vi "movimentacao_cin_inv_bezier_2_com_sensor.vi"() -> ()   [LabVIEW 2017]
doc: "The myRIO Project template acquires acceleration data from the onboard accelerometer and displays the changes of acceleration values in a waveform chart."
uses:
  <vilib>/Analysis/Matrix/Datatypes/RealMatrix.ctl
  <vilib>/myRIO/Instrument Drivers/Onboard IO/I2C/typedefs/I2C User Configuration.ctl
  <vilib>/myRIO/Instrument Drivers/Onboard IO/I2C/typedefs/I2C Transfer Rate.ctl
  <vilib>/myRIO/Instrument Drivers/Onboard IO/PWM/typedefs/PWM Reference.ctl
  <vilib>/myRIO/Common/Instrument Driver Framework/Utilities/typedefs/myRIO Generic Hardware Reference.ctl
  <vilib>/myRIO/Common/Instrument Driver Framework/Utilities/typedefs/Hardware Version Enum.ctl
  <vilib>/myRIO/Common/Instrument Driver Framework/Utilities/typedefs/myRIO v1.0 Reference.ctl
  <vilib>/myRIO/Common/Instrument Driver Framework/Utilities/typedefs/Generic FPGA Reference.ctl
  <vilib>/myRIO/Common/Instrument Driver Framework/myRIO v1.0/PWM/typedefs/PWM Channels Enum.ctl
  <vilib>/myRIO/Instrument Drivers/Onboard IO/PWM/typedefs/PWM Configuration.ctl
  <vilib>/userdefined/High Color/nirio_resource_hc.ctl
  <vilib>/myRIO/Instrument Drivers/Onboard IO/I2C/typedefs/I2C Reference.ctl
  <vilib>/myRIO/Common/Instrument Driver Framework/myRIO v1.0/I2C/typedefs/I2C Channels Enum.ctl
  <vilib>/myRIO/Instrument Drivers/Onboard IO/I2C/typedefs/I2C Configuration.ctl
  <vilib>/myRIO/Common/Instrument Driver Framework/myRIO v1.0/I2C/vis/myRIO v1.1 Open I2C.vi
  <vilib>/myRIO/Common/Instrument Driver Framework/myRIO v1.0/PWM/vis/myRIO v1.1 Open PWM.vi
  <vilib>/myRIO/Common/Instrument Driver Framework/Utilities/vis/Validate Channels.vi
  <vilib>/myRIO/Common/Instrument Driver Framework/myRIO v1.0/I2C/vis/myRIO v1.0 Reserve I2C.vi
  <vilib>/myRIO/Common/Instrument Driver Framework/myRIO v1.0/I2C/vis/myRIO v1.0 Close I2C.vi
  <vilib>/myRIO/Common/Instrument Driver Framework/myRIO v1.0/PWM/vis/myRIO v1.0 Reserve PWM.vi
  <vilib>/myRIO/Instrument Drivers/Onboard IO/PWM/vis/Set Duty Cycle and Frequency.vi
  <vilib>/myRIO/Common/Instrument Driver Framework/myRIO v1.0/PWM/vis/myRIO v1.0 Close PWM.vi
  <vilib>/myRIO/Common/Instrument Driver Framework/myRIO v1.0/I2C/vis/myRIO v1.0 Build MUX Configuration I2C.vi
  <vilib>/myRIO/Common/Instrument Driver Framework/myRIO v1.0/Resource Manager/vis/myRIO v1.0 Reserve Channel List.vi
  <vilib>/myRIO/Common/Instrument Driver Framework/myRIO v1.0/I2C/vis/myRIO v1.0 Unreserve I2C.vi
  <vilib>/myRIO/Common/Instrument Driver Framework/myRIO v1.0/PWM/vis/myRIO v1.0 Build MUX Configuration PWM.vi
  <vilib>/myRIO/Common/Instrument Driver Framework/myRIO v1.0/PWM/vis/myRIO v1.0 Unreserve PWM.vi
  <vilib>/myRIO/Common/Instrument Driver Framework/myRIO v1.0/Resource Manager/vis/myRIO v1.0 Create Configuration List.vi
  <vilib>/myRIO/Common/Instrument Driver Framework/myRIO v1.0/Resource Manager/vis/myRIO v1.0 Reserve Channel.vi
  <vilib>/myRIO/Common/Instrument Driver Framework/myRIO v1.0/Resource Manager/vis/myRIO v1.0 Unreserve Channel.vi
  <vilib>/myRIO/Common/Instrument Driver Framework/myRIO v1.0/Resource Manager/vis/myRIO v1.0 Unreserve Channel List.vi
  <vilib>/myRIO/Common/Instrument Driver Framework/myRIO v1.0/Resource Manager/vis/myRIO v1.0 Build Mutex Name.vi
  <vilib>/Utility/VariantDataType/GetNumericInfo.vi
  <vilib>/Utility/error.llb/Error Cluster From Error Code.vi
  <vilib>/myRIO/Common/Instrument Driver Framework/myRIO v1.0/myRIO v1.1 Open.vi
  <vilib>/myRIO/Common/Instrument Driver Framework/Utilities/vis/IO Manager.vi
  <vilib>/myRIO/Common/Instrument Driver Framework/Utilities/vis/Configuration Manager.vi
  <vilib>/myRIO/Common/Instrument Driver Framework/myRIO v1.0/Resource Manager/vis/myRIO v1.0 Configure IO.vi
  <vilib>/myRIO/Common/Instrument Driver Framework/myRIO v1.0/myRIO v1.0 Close.vi
  <vilib>/myRIO/Common/Instrument Driver Framework/myRIO v1.0/PWM/vis/myRIO v1.0 Write PWM.vi
  <vilib>/myRIO/Common/Instrument Driver Framework/myRIO v1.0/PWM/vis/myRIO v1.0 Shutdown PWM.vi
  <vilib>/myRIO/Common/Instrument Driver Framework/myRIO v1.0/I2C/vis/myRIO v1.0 Configure I2C.vi
  <vilib>/myRIO/Common/Instrument Driver Framework/myRIO v1.0/I2C/vis/myRIO v1.0 Shutdown I2C.vi
  <vilib>/myRIO/Instrument Drivers/Onboard IO/PWM/vis/myRIO PWM Open.xnode
  <vilib>/myRIO/Instrument Drivers/Onboard IO/I2C/vis/myRIO I2C Open.xnode
  <vilib>/myRIO/Instrument Drivers/Onboard IO/PWM/PWM.lvlib
  <vilib>/myRIO/Instrument Drivers/Onboard IO/I2C/I2C.lvlib
  <vilib>/Analysis/Matrix/NI_Matrix.lvlib
panel:
  out "Detectou 2":bool
  out "mean out":dbl
  in  "y":dbl=135.0
  out "PARAR ESTEIRA":bool
  out "reconheceu":bool
  out "Boolean":bool
  out "x .and. y? 2":bool
  out "Detectou":bool
  in  "Duty Cycle Abert 2":dbl=0.08 format="%#_13g"
  out "Local_da_peca":i8
  out "PARAR 2":bool
  out "spreadsheet string":string
  out "error out 2":errorcluster
  out "init status 2":bool
  out "did_timeout 2":bool
  out "dt 2":u32
  out "Waveform Chart 2":u16(graph)
  out "Range (cm)":u16
  out "objeto":bool
  out "distancaia 2":dbl format="%0.2f"
  out "result string":string
  out "iterador":u32
  out "number of rows":i32
  out "matrix":T1
  out "subarray":dbl[](array[numeric])
  out "appended array 2":dbl[](array[numeric])
  out "POS_E_ORIEN_HOME":dbl[](array[numeric])
  out "ANG_POSI_E_ORIEN_HOME":dbl[](array[numeric])
  out "CURRENT POSITIONS OF THE MOTORS":dbl[](array[numeric])
  in  "angulo_garra":dbl(knob) scale=-180.0..180.0
  in  "Duty Cycle Abert":dbl=0.04 format="%#_13g"
  out "Actuator 2":bool
  in  "Actuator":bool
  in  "Conveyor speed (mm/s)":dbl(slide)=200.0 step=1.0 scale=0.0..350.0
  out "indexador":i32
  out "Manipulando":bool
  out "Está em Home":bool
  out "Posicao_desejada":bool
  in  "Home":bool
  in  "error in (no error)":errorcluster
  in  "PARAR":bool
  in  "POSITION VECTOR":dbl[](array[numeric])
  # "ROTINA DE CONTROLE DO PROTÓTIPO DE FMS"
  # "COMANDO DE POSI敲O\nATUAL DOS MOTORES"
  # "OPERATION STATUS"
  # "ÂNGULOS DE JUNTAS"
  # "THETA 1"
  # "MOTOR 1"
  # "HOME"
  # "THETA 2"
  # "MOTOR 2"
  # "POSI敲O DESEJADA"
  # "SCL- CINZA - 32\nSDA - ROXO - 34\nTERRA - BRANCO\nVCC - PRETO"
  # "THETA 3"
  # "MOTOR 3"
  # "OBJETO DETECTADO"
  # "THETA 4"
  # "MOTOR 4"
  # "MANIPULANDO"
  # "THETA 5"
  # "MOTOR 5"
  # "ESTEIRA PARADA"
  # "MOTOR 6"
  # "ATUADOR"
  # "VELOCIDADE DA ESTEIRA (mm/s)"
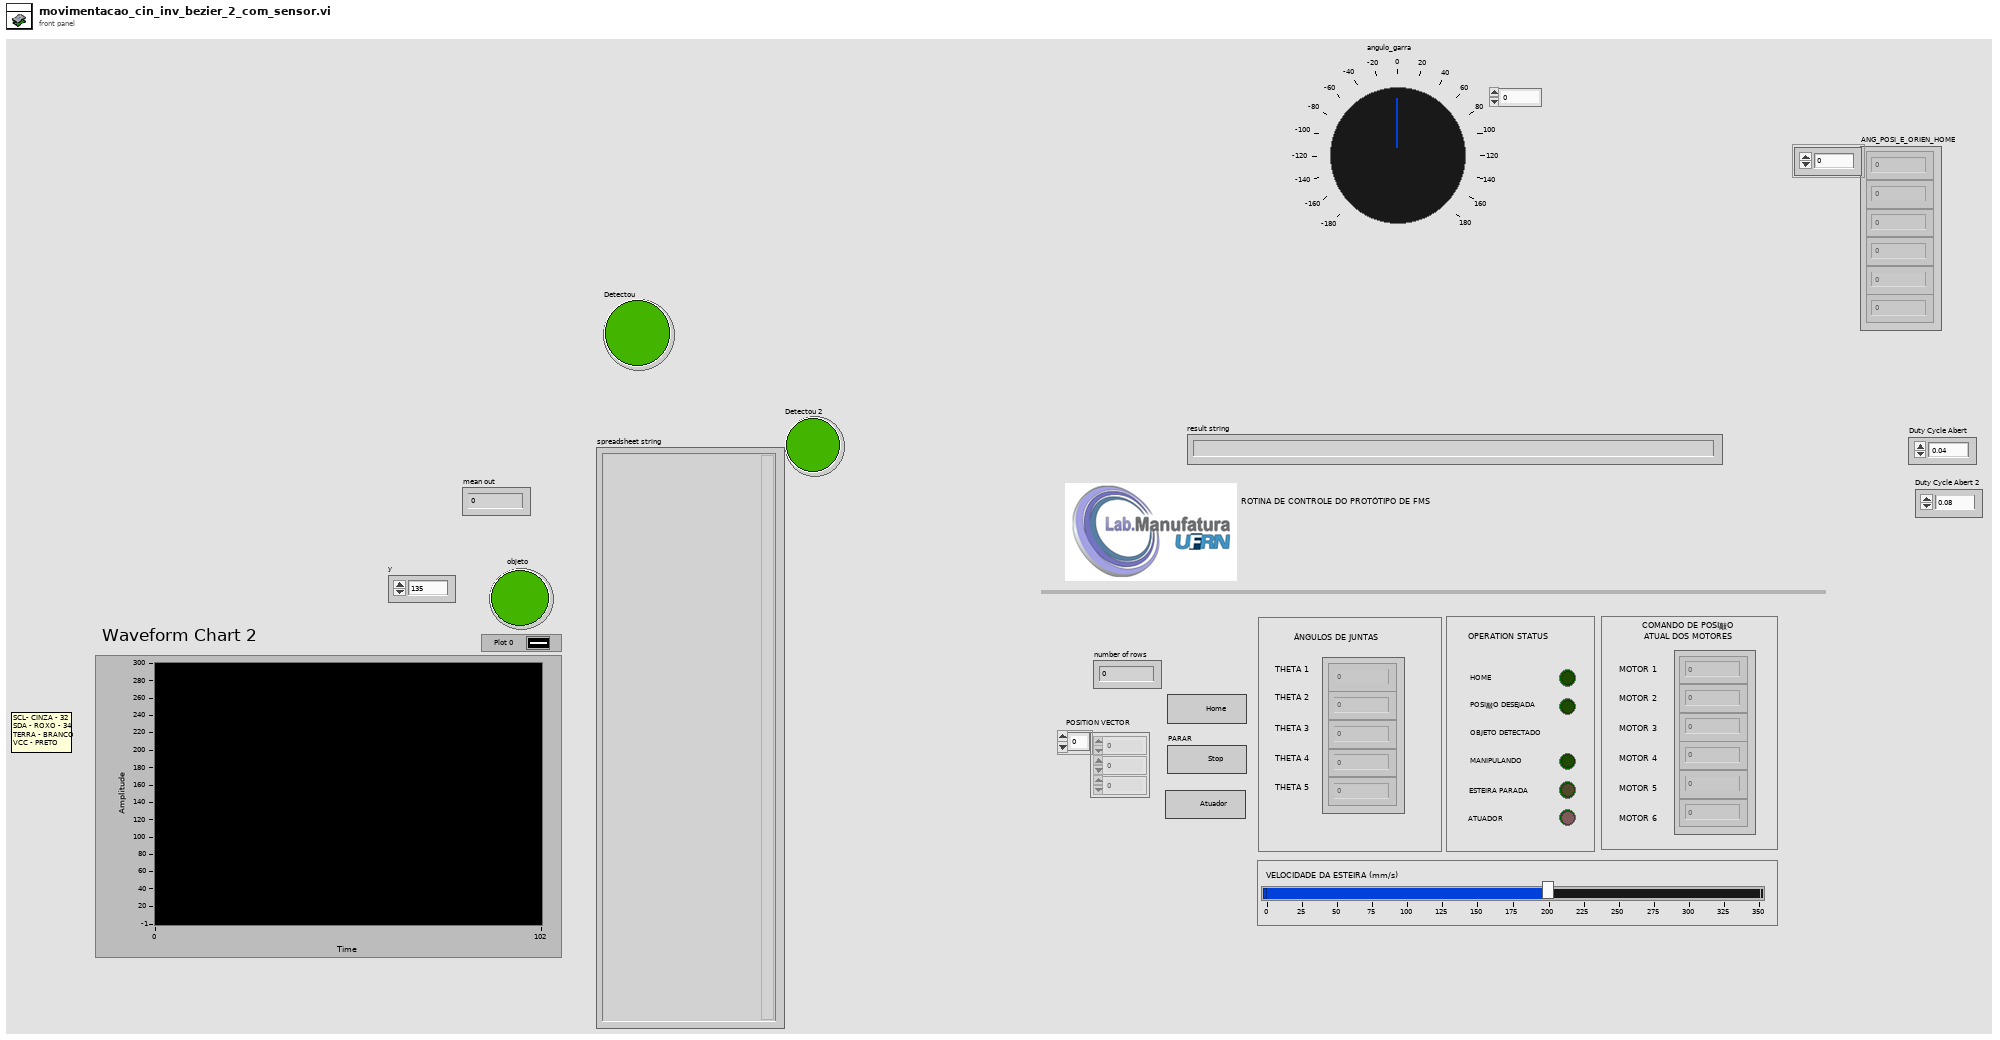
[diagram p1: front panel]
types:
  T1 = typedef "NI_Matrix.lvlib/RealMatrix.ctl" = dbl[][]
  T2 = typedef "I2C.lvlib/I2C User Configuration.ctl" = cluster{"I2C Transfer Rate":T3}
  T3 = typedef "I2C.lvlib/I2C Transfer Rate.ctl" = enum16{"Standard mode (100 kbps)", "Fast mode (400 kbps)"}
  T4 = cluster{"theta 1":dbl, "theta 2":dbl, "theta 3":dbl, "theta5":dbl, "theta4":dbl}
  T5 = typedef "nirio_resource_hc.ctl" = tag
  T6 = typedef "Hardware Version Enum.ctl" = enum16{"Unknown", "myRIO-1900", "myRIO-1950", "roboRIO", "NI ELVIS RIO CM"}
  T7 = typedef "PWM.lvlib/PWM Reference.ctl" = cluster{"myRIO Reference":T8, "PWM Channels Enum":T11, "PWM Configuration":T12}
  T8 = typedef "myRIO Generic Hardware Reference.ctl" = cluster{"myRIO Model":T6, "myRIO Hardware Reference":T9}
  T9 = typedef "myRIO v1.0 Reference.ctl" = cluster{"Generic FPGA Reference":T10, "Allow multiple opens":bool}
  T10 = typedef "Generic FPGA Reference.ctl" = refnum<k20>
  T11 = typedef "PWM Channels Enum.ctl" = enum16{"Not Connected", "C/PWM0", "C/PWM1", "A/PWM0", "A/PWM1", "A/PWM2", "B/PWM0", "B/PWM1", "B/PWM2", "PWM/PWM0", "PWM/PWM1", "PWM/PWM2", "PWM/PWM3", "PWM/PWM4", "PWM/PWM5", "PWM/PWM6", "PWM/PWM7", "PWM/PWM8", "PWM/PWM9"}
  T12 = typedef "PWM.lvlib/PWM Configuration.ctl" = cluster{"Frequency":dbl, "Duty Cycle":dbl}
  T13 = typedef "I2C.lvlib/I2C Reference.ctl" = cluster{"myRIO Reference":T8, "I2C Channels Enum":T14, "I2C Configuration":T15}
  T14 = typedef "I2C Channels Enum.ctl" = enum16{"Not Connected", "A/I2C", "B/I2C", "I2C/I2C"}
  T15 = typedef "I2C.lvlib/I2C Configuration.ctl" = cluster{"I2C Transfer Rate":T3}
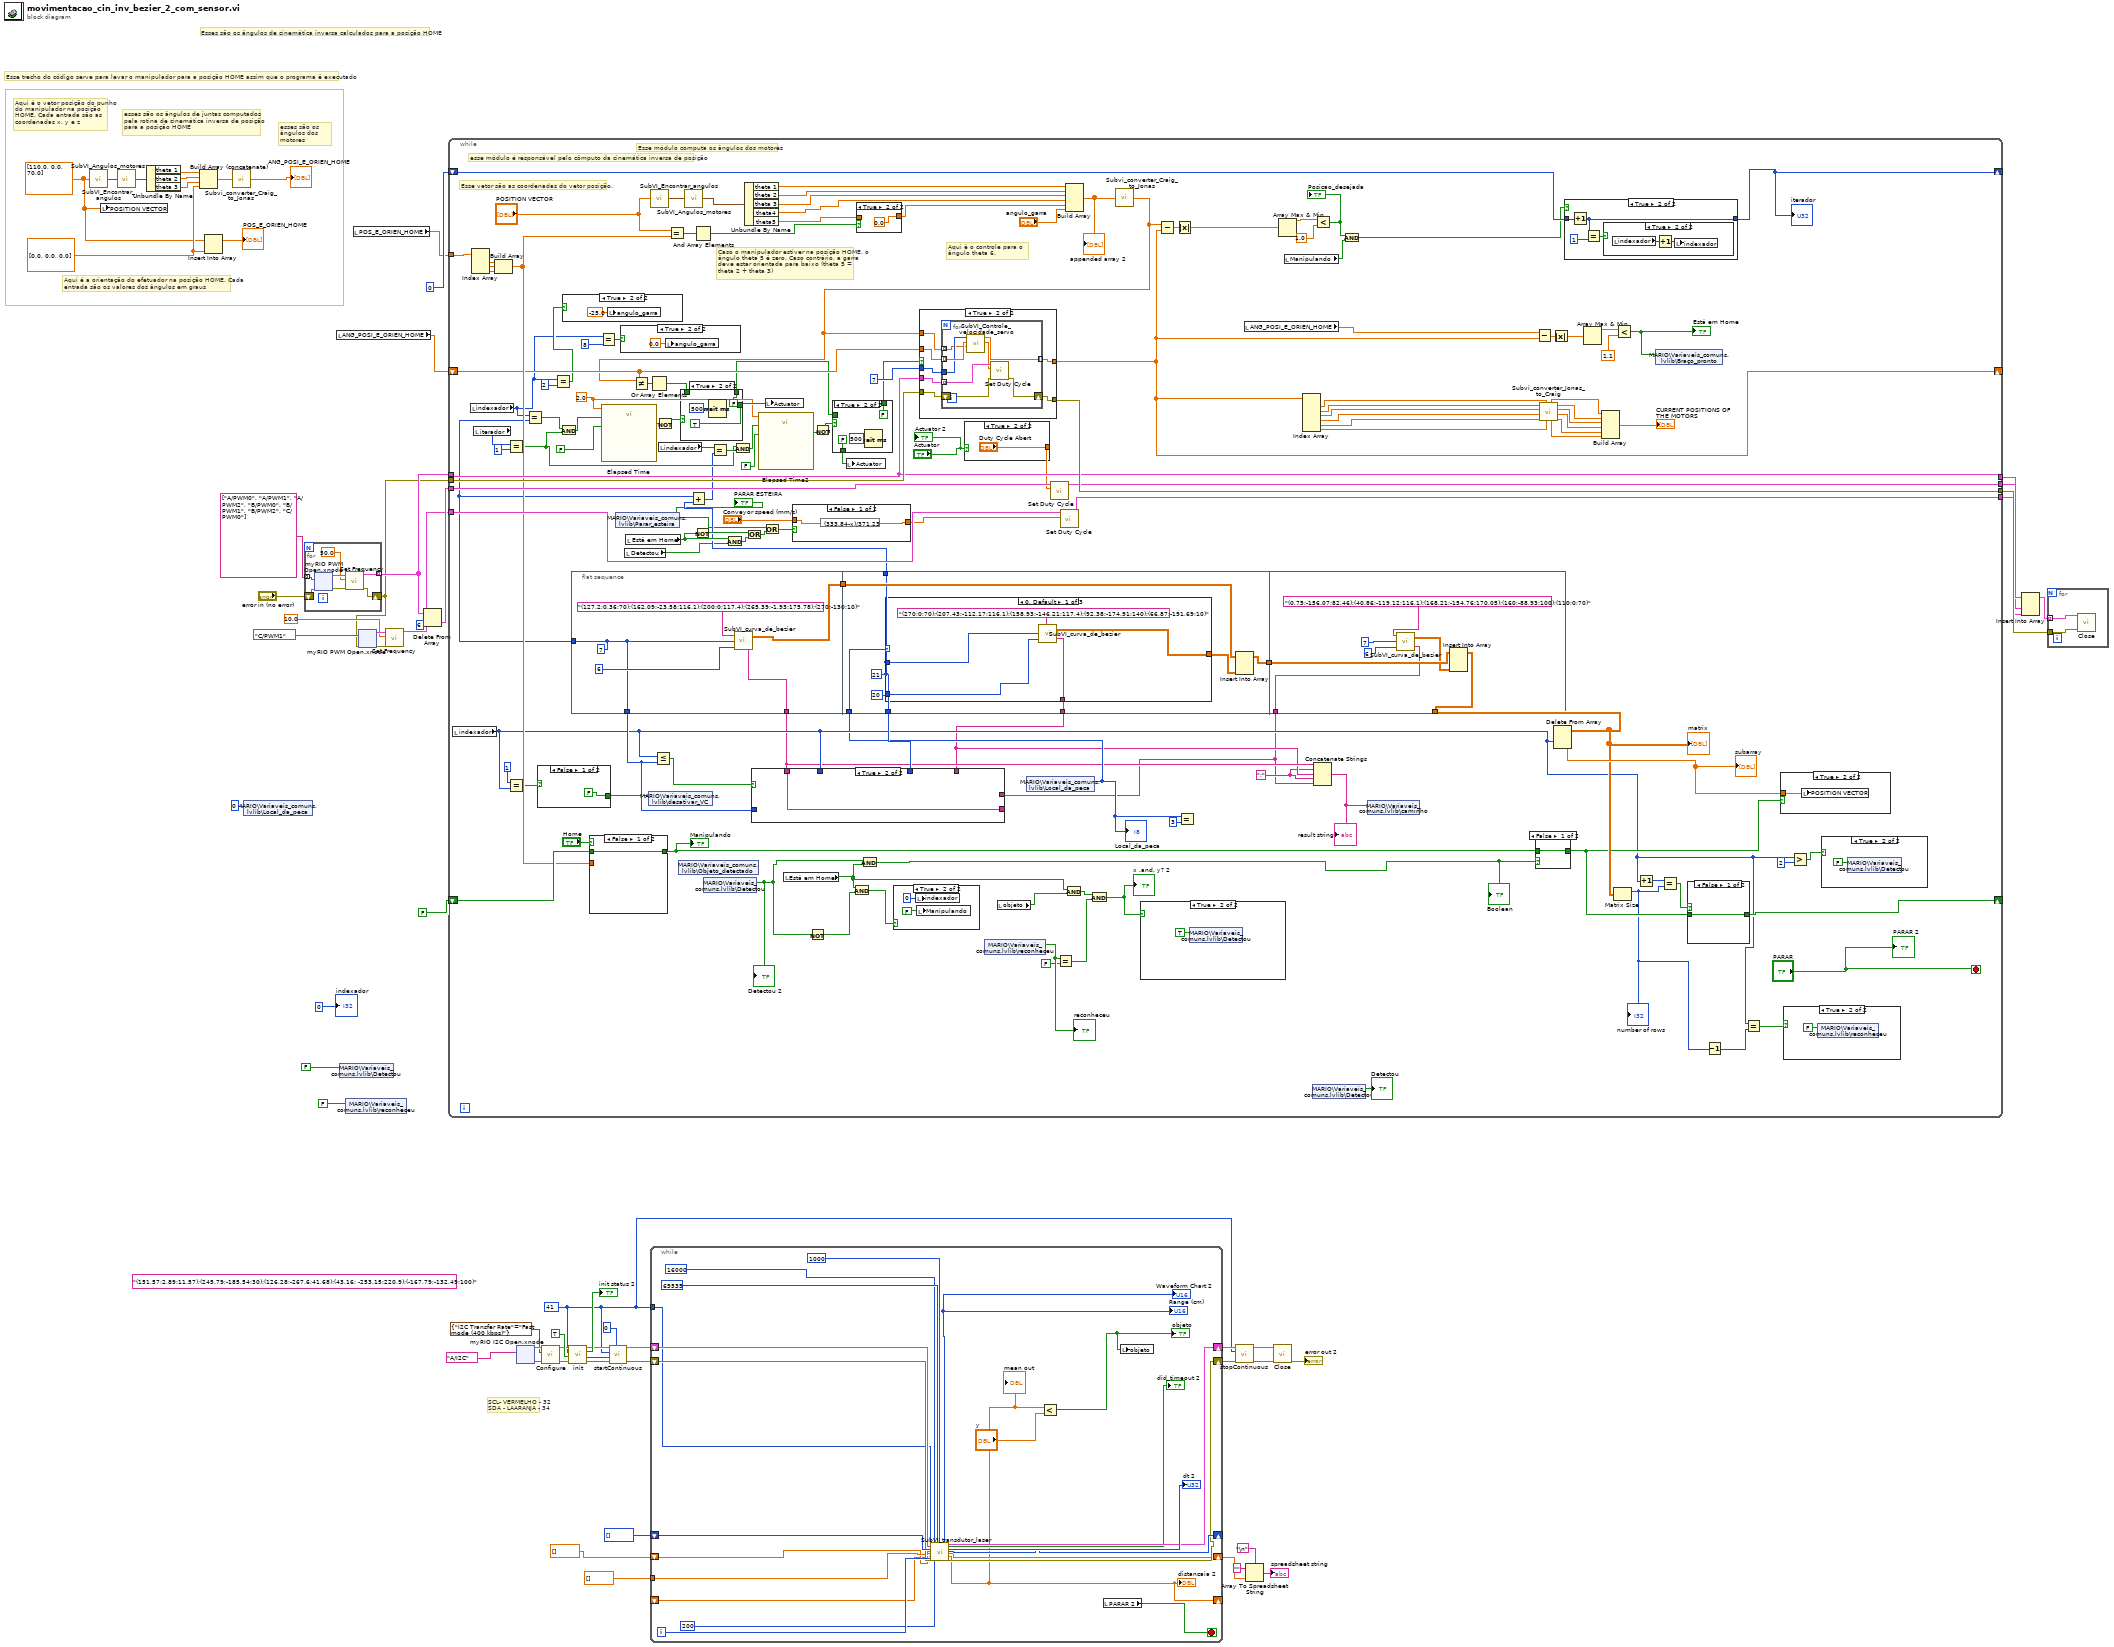
[diagram p0: block diagram]
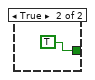
[diagram p5: hidden frame]
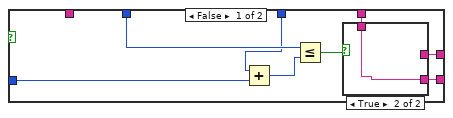
[diagram p8: hidden frame]
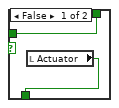
[diagram p10: hidden frame]
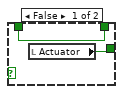
[diagram p11: hidden frame]
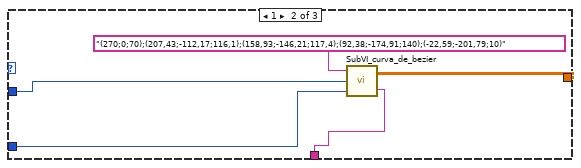
[diagram p13: hidden frame]
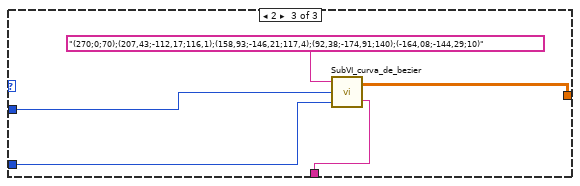
[diagram p14: hidden frame]
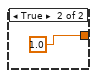
[diagram p15: hidden frame]
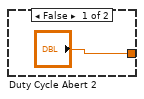
[diagram p16: hidden frame]
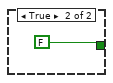
[diagram p18: hidden frame]
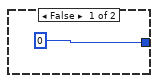
[diagram p19: hidden frame]
diagram:
  w11 = u8 41
  (unwired) "(151,57;2,89;11,57);(245,79;-185,54;30);(126,28;-267,6;41,68);(43,16; -253,15;220,9);(-167,79;-132,49;100)" ("String 2")
  w38 = dbl[] [0.0, 0.0, 0.0] ("vetor_P")
  w1 = dbl[] [110.0, 0.0, 70.0] ("vetor_P")
  # "esses são os ângulos dos motores"
  # "esses são os ângulos de juntas computados pela rotina de cinemática inversa de posição para a posição HOME"
  # "Esses são os ângulos de cinemática inversa calculados para a posição HOME"
  # "Aqui é a orientação do efetuador na posição HOME. Cada entrada são os valores dos ângulos em graus"
  # "Aqui é o vetor posição do punho do manipulador na posição HOME. Cada entrada são as coordenadas x, y e z"
  # "Esse trecho do código serve para levar o manipulador para a posição HOME assim que o programa é executado"
  # "SCL- VERMELHO - 32\nSDA - LAARANJA - 34"
  n1 = call "SubVI_Encontrar_angulos.vi"("vetor_P"=w1) -> ("ângulos de Juntas"=w33:T4)
  n2 = local write "POSITION VECTOR"(w1) -> ()
  n3 = call "SubVI_Angulos_motores.vi"("input cluster"=w33) -> ("output cluster"=w32:T4)
  n4 = Unbundle By Name(w32) -> ("theta 1"=w42:dbl, "theta 2"=w41:dbl, "theta 3"=w40:dbl)
  n5 = Build Array (concatenate)(w42, w41, w40, w38) -> (w35:dbl[])
  n6 = Insert Into Array(array=w1, new element=w38) -> (→"POS_E_ORIEN_HOME":dbl[])  [unwired: 1 in]
  n7 = call "Subvi_converter_Craig_to_Jonas.vi"("array"=w35) -> ("appended array"=→"ANG_POSI_E_ORIEN_HOME":dbl[])
  n8 = shared-variable "MARIO\\Variaveis_comuns.lvlib\\Local_da_peca"(i8 0 ("Local_da_peca")) -> ()  [unwired: 1 in, 1 out]
  n9 = for {
    tunnel: tag[] ["A/PWM0", "A/PWM1", "A/PWM2", "B/PWM0", "B/PWM1", "B/PWM2", "C/PWM0"] -> [w65] mode=indexing
    tunnel: [w64] -> w55 mode=indexing
    shift-right: [w63] -> w44
    shift-left: "error in (no error)" -> [w62]
    n10 = xnode ("myRIO PWM Open.xnode")("error in (no error)"=w62, "Channel Name"=w65) -> ("error out"=w66:errorcluster, "PWM Ref Out"=w68:T7)  [unwired: 1 in]
    n11 = call <vilib>:"Set Frequency.vi"("error in (no error)"=w66, "Frequency [Hz]"=50.0, "PWM Ref In"=w68) -> ("error out"=w63:errorcluster, "PWM Ref Out"=w64:T7)  [unwired: 6 in]
  }
  n12 = local read "ANG_POSI_E_ORIEN_HOME"() -> (w39:dbl[])
  n13 = shared-variable "MARIO\\Variaveis_comuns.lvlib\\Detectou"(FALSE ("Detectou")) -> ()  [unwired: 1 in, 1 out]
  n14 = shared-variable "MARIO\\Variaveis_comuns.lvlib\\reconheceu"(FALSE ("reconheceu")) -> ()  [unwired: 1 in, 1 out]
  n15 = local read "POS_E_ORIEN_HOME"() -> (w36:dbl[])
  n16 = xnode "myRIO PWM Open.xnode"("error in (no error)"=w44, "Channel Name"=tag "C/PWM1") -> ("error out"=w48:errorcluster, "PWM Ref Out"=w49:T7)  [unwired: 1 in]
  n17 = call <vilib>:"Set Frequency.vi"("error in (no error)"=w48, "Frequency [Hz]"=10.0, "PWM Ref In"=w49) -> ("PWM Ref Out"=w45:T7)  [unwired: 6 in, 1 out]
  n18 = Delete From Array(array=w55, index=6) -> (deleted portion=w53:T7)  [unwired: 1 in, 1 out]
  n19 = while {
    tunnel: [w223] -> w61
    shift-right: [w161] -> _
    shift-left: w39 -> [w153]
    tunnel: w44 -> [w221]
    tunnel: w55 -> [w220]
    tunnel: [w220] -> w52
    shift-right: [w148] -> _
    shift-left: FALSE -> [w205]
    shift-right: [w214] -> _
    shift-left: u32 0 ("ms to wait (braço)") -> [w213]
    tunnel: w53 -> [w200]
    tunnel: [w199] -> w51
    tunnel: w45 -> [w197]
    tunnel: [w193] -> w43
    tunnel: w36 -> [w166]
    stop <- "PARAR" stop-if-true
    w87 = ";" ("string")
    w132 = 2.0 ("Time Target (s)")
    # "Aqui é o controle para o ângulo theta 6."
    # "Caso o manipulador estiver na posição HOME, o ângulo theta 5 é zero. Caso contrário, a garra deve estar orientada para baixo (theta 5 = theta 2 + theta 3)"
    # "Esse módulo computa os ângulos dos motores"
    # "esse módulo é responsável pelo cômputo da cinemática inversa de posição"
    # "Esse vetor são as coordenadas do vetor posição."
    n20 = local read "indexador"() -> (w100:i32)
    n21 = local read "indexador"() -> (w115:i32)
    n22 = Index Array(array=w166) -> (element #1=w169:dbl, element #2=w168:dbl, element #3=w167:dbl)  [unwired: 3 in]
    n23 = local read "iterador"() -> (w145:u32)
    n24 = Build Array(w169, w168, w167) -> (w165:dbl[])
    n25 = Equal?(x=w145, y=u32 1) -> (x = y?=w134:bool)
    n26 = Equal?(x=1, y=w100) -> (x = y?=w113:bool)
    n27 = Equal?(x=w115, y=w123) -> (x = y?=w137:bool)
    n28 = case shown="False" w113 {
      tunnel: [FALSE TRUE] -> w112
      frame False {
      }
      frame True {
      }
    }
    n29 = Equal?(x=w115, y=2) -> (x = y?=w118:bool)
    n30 = And(x=w137, y=w134) -> (x .and. y?=w143:bool)
    n31 = case shown="True" w118 {
      frame False {
      }
      frame True {
        n32 = local write "angulo_garra"(-25.0 ("angulo_garra")) -> ()
      }
    }
    n33 = flat-sequence {
      tunnel: [w257] -> w151
      tunnel: [w255] -> w123
      tunnel: [w255] -> w120
      tunnel: [w254] -> w89
      tunnel: w151 -> [w264]
      tunnel: [w265] -> w150
      tunnel: [w260] -> w124
      tunnel: w95 -> [w261]
      tunnel: [w260] -> w121
      tunnel: [w259] -> w88
      tunnel: [w282] -> w149
      tunnel: w150 -> [w284]
      tunnel: [w281] -> w86
      frame #0 {
        w255 = i64 7 ("número de pontos que a matriz deve retornar (nº de divisões + 1)")
        n34 = call "SubVI_curva_de_bezier.vi"("Nº de divisões da curva de Bézier (padrão: 20 divisões = 21 pontos)"=6, "número de pontos que a matriz deve retornar (padrão: nº de divisões + 1)"=w255, "String in"="(127,2;0,36;70);(162,09;-23,58;116,1);(200;0;117,4);(265,39;-1,93;175,78);(270;-130;10)" ("Esteira")) -> ("result string"=w254:string, "matrix"=w257:T1)
      }
      frame #1 {
        w260 = i64 21 ("número de pontos que a matriz deve retornar (nº de divisões + 1)")
        n35 = case shown="0, Default" w261 {
          tunnel: [w270 w275 w280] -> w263
          tunnel: w260 -> [w268 w274 w278]
          tunnel: 20 ("Nº de divisões da curva de Bézier (padrão: 20 divisões = 21 pontos)") -> [w267 w273 w277]
          tunnel: [w266 w271 w276] -> w259
          frame 0, Default {
            n36 = call "SubVI_curva_de_bezier.vi"("Nº de divisões da curva de Bézier (padrão: 20 divisões = 21 pontos)"=w267, "número de pontos que a matriz deve retornar (padrão: nº de divisões + 1)"=w268, "String in"="(270;0;70);(207,43;-112,17;116,1);(158,93;-146,21;117,4);(92,38;-174,91;140);(66,87;-191,69;10)" ("Esteira")) -> ("result string"=w266:string, "matrix"=w270:T1)
          }
          frame 1 {
            n37 = call "SubVI_curva_de_bezier.vi"("Nº de divisões da curva de Bézier (padrão: 20 divisões = 21 pontos)"=w273, "número de pontos que a matriz deve retornar (padrão: nº de divisões + 1)"=w274, "String in"="(270;0;70);(207,43;-112,17;116,1);(158,93;-146,21;117,4);(92,38;-174,91;140);(-22,59;-201,79;10)" ("Esteira")) -> ("result string"=w271:string, "matrix"=w275:T1)
          }
          frame 2 {
            n38 = call "SubVI_curva_de_bezier.vi"("Nº de divisões da curva de Bézier (padrão: 20 divisões = 21 pontos)"=w277, "número de pontos que a matriz deve retornar (padrão: nº de divisões + 1)"=w278, "String in"="(270;0;70);(207,43;-112,17;116,1);(158,93;-146,21;117,4);(92,38;-174,91;140);(-164,08;-144,29;10)" ("Esteira")) -> ("result string"=w276:string, "matrix"=w280:T1)
          }
        }
        n39 = Insert Into Array(array=w264, new element=w263) -> (w265:T1)  [unwired: 2 in]
      }
      frame #2 {
        n40 = call "SubVI_curva_de_bezier.vi"("Nº de divisões da curva de Bézier (padrão: 20 divisões = 21 pontos)"=6, "número de pontos que a matriz deve retornar (padrão: nº de divisões + 1)"=i64 7 ("número de pontos que a matriz deve retornar (nº de divisões + 1)"), "String in"="(0,75;-156,07;82,46);(40,86;-119,12;116,1);(168,21;-154,76;170,05);(160;-88,93;100);(110;0;70)" ("Esteira")) -> ("result string"=w281:string, "matrix"=w283:T1)
        n41 = Insert Into Array(array=w284, new element=w283) -> (w282:T1)  [unwired: 2 in]
      }
    }
    n42 = case shown="False" "Home" {
      tunnel: w165 -> [_ w312]
      tunnel: w205 -> [w308 _]
      tunnel: [w308 FALSE ("Manipulando")] -> w160
      frame False {
      }
      frame True {
        n43 = local write "POSITION VECTOR"(w312) -> ()
        n44 = local write "angulo_garra"(0.0 ("angulo_garra")) -> ()
        n45 = local write "indexador"(0 ("indexador")) -> ()
      }
    }
    "Manipulando" <- w160
    n46 = Equal?(x=w115, y=8) -> (x = y?=w116:bool)
    n47 = call "Elapsed Time"("Time Target (s)"=w132, "Reset"=w143, "Auto Reset"=FALSE) -> ("Time has Elapsed"=w141:bool)  [unwired: 9 in, 7 out]
    n48 = shared-variable "MARIO\\Variaveis_comuns.lvlib\\Parar_esteira"() -> (w94:bool)  [unwired: 1 in, 1 out]
    "PARAR ESTEIRA" <- w94
    n49 = case shown="True" w116 {
      frame False {
      }
      frame True {
        n50 = local write "angulo_garra"(0.0 ("angulo_garra")) -> ()
      }
    }
    n51 = local read "Detectou"() -> (w92:bool)
    n52 = local read "Está em Home"() -> (w189:bool)
    n53 = shared-variable "MARIO\\Variaveis_comuns.lvlib\\desativar_VC"(w112) -> ()  [unwired: 1 in, 1 out]
    n54 = call "SubVI_Encontrar_angulos.vi"("vetor_P"="POSITION VECTOR") -> ("ângulos de Juntas"=w158:T4)
    n55 = Less Or Equal?(x=w100, y=w120) -> (x <= y?=w122:bool)
    n56 = Not(x=w141) -> (.not. x?=w140:bool)
    n57 = local read "indexador"() -> (w136:i32)
    n58 = Equal?(x="POSITION VECTOR", y=w165) -> (x = y?=w203:bool[])
    n59 = shared-variable "MARIO\\Variaveis_comuns.lvlib\\Objeto_detectado"() -> ()  [unwired: 1 in, 2 out]
    n60 = call "SubVI_Angulos_motores.vi"("input cluster"=w158) -> ("output cluster"=w157:T4)
    n61 = Add(x=w123, y=w124) -> (x+y=w125:i64)
    n62 = Not(x=w189) -> (.not. x?=w190:bool)
    n63 = And Array Elements(Boolean array=w203) -> (logical AND=w202:bool)
    n64 = shared-variable "MARIO\\Variaveis_comuns.lvlib\\Detectou"() -> (w93:bool)  [unwired: 1 in, 1 out]
    "Detectou 2" <- w93
    n65 = Equal?(x=w136, y=w125) -> (x = y?=w135:bool)
    n66 = And(x=w189, y=w92) -> (x .and. y?=w191:bool)
    n67 = And(x=w134, y=w135) -> (x .and. y?=w133:bool)
    n68 = Unbundle By Name(w157) -> ("theta 1"=w174:dbl, "theta 2"=w173:dbl, "theta 3"=w172:dbl, "theta4"=w156:dbl, "theta5"=w155:dbl)
    n69 = Or(x=w190, y=w191) -> (x .or. y?=w188:bool)
    n70 = case shown="True" w122 {
      tunnel: w89 -> [_ w242]
      tunnel: w100 -> [w239 _]
      tunnel: w121 -> [w234 _]
      tunnel: [w237 w242] -> _
      tunnel: w88 -> [w236 _]
      tunnel: w86 -> [w235 _]
      tunnel: w120 -> [w233 _]
      frame False {
        n71 = Add(x=w234, y=w233) -> (x+y=w232:i64)
        n72 = Less Or Equal?(x=w239, y=w232) -> (x <= y?=w238:bool)
        n73 = case shown="True" w238 {
          tunnel: [w240 w241] -> w237
          tunnel: w236 -> [_ w241]
          tunnel: w235 -> [w240 _]
          frame False {
          }
          frame True {
          }
        }
      }
      frame True {
      }
    }
    n74 = call "Elapsed Time2"("Time Target (s)"=w132, "Reset"=w133, "Auto Reset"=FALSE) -> ("Time has Elapsed"=w131:bool)  [unwired: 9 in, 7 out]
    n75 = Or(x=w94, y=w188) -> (x .or. y?=w194:bool)
    n76 = local read "Está em Home"() -> (w111:bool)
    n77 = case shown="False" w194 {
      tunnel: [w289 1.0 ("Duty Cycle")] -> w196
      tunnel: "Conveyor speed (mm/s)" -> [w288 _]
      frame False {
        n78 = expression code="(333.84-x)/371.23"(w288) -> (w289:dbl)
      }
      frame True {
      }
    }
    n79 = Not(x=w93) -> (.not. x?=w163:bool)
    n80 = Not(x=w131) -> (.not. x?=w130:bool)
    n81 = And(x=w111, y=w163) -> (x .and. y?=w210:bool)
    n82 = case shown="True" w202 {
      tunnel: [w293 0.0 ("theta5")] -> w171
      tunnel: w155 -> [w293 _]
      frame False {
      }
      frame True {
      }
    }
    n83 = And(x=w93, y=w111) -> (x .and. y?=w96:bool)
    "Boolean" <- w96
    n84 = case shown="True" w210 {
      frame False {
      }
      frame True {
        n85 = local write "indexador"(0 ("indexador")) -> ()
        n86 = local write "Manipulando"(FALSE ("Manipulando")) -> ()
      }
    }
    n87 = case shown="True" "Actuator" {
      tunnel: ["Duty Cycle Abert 2" "Duty Cycle Abert"] -> w198
      frame False {
      }
      frame True {
      }
    }
    n88 = shared-variable "MARIO\\Variaveis_comuns.lvlib\\reconheceu"() -> (w108:bool)  [unwired: 1 in, 1 out]
    "reconheceu" <- w108
    n89 = local read "objeto"() -> (w110:bool)
    n90 = shared-variable "MARIO\\Variaveis_comuns.lvlib\\Local_da_peca"() -> (w95:i8)  [unwired: 1 in, 1 out]
    "Local_da_peca" <- w95
    n91 = call <vilib>:"Set Duty Cycle.vi"("Duty Cycle"=w198, "PWM Ref In"=w200) -> ("PWM Ref Out"=w199:T7)  [unwired: 7 in, 1 out]
    n92 = Equal?(x=w108, y=FALSE) -> (x = y?=w106:bool)
    n93 = call <vilib>:"Set Duty Cycle.vi"("Duty Cycle"=w196, "PWM Ref In"=w197) -> ("PWM Ref Out"=w193:T7)  [unwired: 7 in, 1 out]
    n94 = And(x=w111, y=w110) -> (x .and. y?=w109:bool)
    n95 = Build Array(w174, w173, w172, w156, w171, "angulo_garra") -> (w91:dbl[])
    "appended array 2" <- w91
    n96 = And(x=w109, y=w106) -> (x .and. y?=w105:bool)
    "x .and. y? 2" <- w105
    n97 = call "Subvi_converter_Craig_to_Jonas.vi"("array"=w91) -> ("appended array"=w90:dbl[])
    n98 = Not Equal?(x=w90, y=w153) -> (x != y?=w219:bool[])
    n99 = Or Array Elements(Boolean array=w219) -> (logical OR=w139:bool)
    n100 = case shown="True" w140 {
      tunnel: [w249 FALSE] -> w128
      tunnel: w139 -> [w249 _]
      tunnel: [w248 TRUE ("Actuator")] -> w138
      frame False {
        n101 = local read "Actuator"() -> (w248:bool)
      }
      frame True {
        n102 = Wait (ms)(milliseconds to wait=u32 500) -> ()  [unwired: 1 out]
      }
    }
    n103 = local write "Actuator"(w138) -> ()
    n104 = case shown="True" w130 {
      tunnel: [w244 FALSE ("Actuator")] -> w129
      tunnel: w128 -> [w243 _]
      tunnel: [w243 FALSE] -> w127
      frame False {
        n105 = local read "Actuator"() -> (w244:bool)
      }
      frame True {
        n106 = Wait (ms)(milliseconds to wait=u32 500) -> ()  [unwired: 1 out]
      }
    }
    n107 = local write "Actuator"(w129) -> ()
    n108 = case shown="True" w127 {
      tunnel: [w313 w321] -> w223
      tunnel: w221 -> [w313 w320]
      tunnel: w220 -> [_ w319]
      tunnel: w153 -> [w314 w318]
      tunnel: [w314 w316] -> w161
      tunnel: u32 7 ("ms to wait (braço)") -> [_ w317]
      tunnel: w90 -> [_ w315]
      frame False {
      }
      frame True {
        n109 = for {
          tunnel: w319 -> [w327] mode=indexing
          tunnel: w318 -> [w326] mode=indexing
          tunnel: w317 -> [w324]
          tunnel: [w323] -> w316 mode=indexing
          tunnel: w315 -> [w322] mode=indexing
          shift-right: [w329] -> w321
          shift-left: w320 -> [w328]
          n110 = call "SubVI_Controle_velocidade_servo.vi"("Posição Desejada"=w322, "Posição"=w326, "milliseconds to wait"=w324) -> ("Duty Cycle"=w325:dbl, "Posição"=w323:dbl)  [unwired: 7 in]
          n111 = call <vilib>:"Set Duty Cycle.vi"("error in (no error)"=w328, "Duty Cycle"=w325, "PWM Ref In"=w327) -> ("error out"=w329:errorcluster)  [unwired: 6 in, 1 out]
        }
      }
    }
    n112 = case shown="True" w105 {
      frame False {
      }
      frame True {
        n113 = shared-variable "MARIO\\Variaveis_comuns.lvlib\\Detectou"(TRUE ("Detectou")) -> ()  [unwired: 1 in, 1 out]
      }
    }
    n114 = Subtract(x=w90, y=w161) -> (x-y=w218:dbl[])
    n115 = Absolute Value(x=w218) -> (abs(x)=w217:dbl[])
    n116 = Equal?(x=w95, y=i8 3) -> ()  [unwired: 1 out]
    n117 = local read "ANG_POSI_E_ORIEN_HOME"() -> (w170:dbl[])
    n118 = Array Max & Min(array=w217) -> (max value=w164:dbl)  [unwired: 3 out]
    n119 = local read "Manipulando"() -> (w212:bool)
    n120 = Index Array(array=w161) -> (element #1=w187:dbl, element #2=w186:dbl, element #3=w185:dbl, element #4=w184:dbl, element #5=w183:dbl, element #6=w182:dbl)  [unwired: 6 in]
    n121 = shared-variable "MARIO\\Variaveis_comuns.lvlib\\Detectou"() -> (→"Detectou":bool)  [unwired: 1 in, 1 out]
    n122 = Concatenate Strings(w89, w87, w88, w87, w86) -> (w85:string)
    "result string" <- w85
    n123 = Less?(x=w164, y=1.0) -> (x < y?=w162:bool)
    "Posicao_desejada" <- w162
    n124 = And(x=w162, y=w212) -> (x .and. y?=w211:bool)
    n125 = shared-variable "MARIO\\Variaveis_comuns.lvlib\\caminho"(w85) -> ()  [unwired: 1 in, 1 out]
    n126 = case shown="False" w96 {
      tunnel: [w306 TRUE] -> w146
      tunnel: w160 -> [w306 _]
      frame False {
      }
      frame True {
      }
    }
    n127 = Subtract(x=w170, y=w161) -> (x-y=w209:dbl[])
    n128 = call "Subvi_converter_Jonas_to_Craig.vi"("theta6Jonas"=w182, "theta1Jonas"=w187, "theta5Jonas"=w183, "theta4Jonas"=w184, "theta3Jonas"=w185, "theta2Jonas"=w186) -> ("theta5Craig"=w177:dbl, "theta4Craig"=w178:dbl, "theta3Craig"=w179:dbl, "theta2Craig"=w180:dbl, "theta6Craig"=w176:dbl, "theta1Craig"=w181:dbl)
    n129 = Absolute Value(x=w209) -> (abs(x)=w208:dbl[])
    n130 = Delete From Array(array=w149, index (row)=w100) -> (deleted portion=w152:dbl[])  [unwired: 2 in, 1 out]
    "subarray" <- w152
    n131 = case shown="True" w211 {
      tunnel: w213 -> [_ w301]
      tunnel: [u32 0 ("ms to wait (braço)") w300] -> w214
      frame False {
      }
      frame True {
        n132 = Increment(x=w301) -> (x+1=w300:u32)
        n133 = Equal?(x=w300, y=u32 1) -> (x = y?=w298:bool)
        n134 = case shown="True" w298 {
          frame False {
          }
          frame True {
            n135 = local read "indexador"() -> (w303:i32)
            n136 = Increment(x=w303) -> (x+1=w302:i32)
            n137 = local write "indexador"(w302) -> ()
          }
        }
      }
    }
    "iterador" <- w214
    n138 = Array Max & Min(array=w208) -> (max value=w207:dbl)  [unwired: 3 out]
    n139 = Build Array(w181, w180, w179, w178, w177, w176) -> (→"CURRENT POSITIONS OF THE MOTORS":dbl[])
    n140 = Matrix Size(0:w149) -> (1:w103:i32)  [unwired: 1 out]
    "number of rows" <- w103
    n141 = Less?(x=w207, y=1.1) -> (x < y?=w192:bool)
    "Está em Home" <- w192
    n142 = Increment(x=w100) -> (x+1=w147:i32)
    n143 = shared-variable "MARIO\\Variaveis_comuns.lvlib\\Braço_pronto"(w192) -> ()  [unwired: 1 in, 1 out]
    n144 = Equal?(x=w147, y=w103) -> (x = y?=w204:bool)
    n145 = case shown="False" w204 {
      tunnel: [w295 FALSE ("Manipulando")] -> w148
      tunnel: w146 -> [w295 _]
      frame False {
      }
      frame True {
      }
    }
    n146 = Decrement(x=w103) -> (x-1=w102:i32)
    n147 = Equal?(x=w100, y=w102) -> (x = y?=w101:bool)
    n148 = case shown="True" w146 {
      tunnel: w152 -> [_ w253]
      frame False {
      }
      frame True {
        n149 = local write "POSITION VECTOR"(w253) -> ()
      }
    }
    n150 = case shown="True" w101 {
      frame False {
      }
      frame True {
        n151 = shared-variable "MARIO\\Variaveis_comuns.lvlib\\reconheceu"(FALSE ("reconheceu")) -> ()  [unwired: 1 in, 1 out]
      }
    }
    n152 = Greater?(x=w100, y=2) -> (0:w98:bool)
    n153 = case shown="True" w98 {
      frame False {
      }
      frame True {
        n154 = shared-variable "MARIO\\Variaveis_comuns.lvlib\\Detectou"(FALSE ("Detectou")) -> ()  [unwired: 1 in, 1 out]
      }
    }
    "Actuator 2" <- "Actuator"
    "matrix" <- w149
    "PARAR 2" <- "PARAR"
  }
  n155 = xnode "myRIO I2C Open.xnode"("Channel Name"=tag "A/I2C") -> ("error out"=w30:errorcluster, "I2C Ref Out"=w31:T13)  [unwired: 2 in]
  n156 = call <vilib>:"Configure.vi"("error in (no error)"=w30, "I2C User Configuration"=T2 {"I2C Transfer Rate"=enum."Fast mode (400 kbps)"}, "I2C Ref In"=w31) -> ("error out"=w21:errorcluster, "I2C Ref Out"=w22:T13)  [unwired: 7 in]
  n157 = call "init.vi"("error in"=w21, "io_2V8"=TRUE, "Slave Address(7 bit)"=w11, "I2C Ref In"=w22) -> ("error out"=w18:errorcluster, "stop_variable"=w17:u8, "Boolean"=→"init status 2":bool, "I2C Ref Out"=w19:T13)  [unwired: 4 in]
  n158 = call "startContinuous.vi"("period_ms"=u32 0, "error in"=w18, "stop_variable"=w17, "Slave Address(7 bit)"=w11, "I2C Ref In"=w19) -> ("error out"=w25:errorcluster, "I2C Ref Out"=w24:T13)  [unwired: 5 in]
  n159 = while {
    shift-right: [w344] -> w15
    shift-left: w24 -> [w346]
    shift-right: [w343] -> w14
    shift-left: w25 -> [w345]
    tunnel: w11 -> [w341]
    shift-right: [w348] -> _
    shift-left: u16[] [] -> [w349]
    tunnel: dbl[] [] ("array") -> [w337]
    shift-right: [w335] -> w6
    shift-left: dbl[] [] ("array") -> [w336]
    shift-right: [w332] -> _
    shift-left: _ -> [w334]
    i -> [w347]
    stop <- w333 stop-if-true
    n160 = call "SubVI_transdutor_laser.vi"("Numeric Control 2"=w341, "I2C Ref Out in"=w346, "Array in"=w349, "array in"=w336, "array 3"=w337, "mean in"=w334, "Numeric Control 3"=w347, "error in (no error)"=w345, "io_timeout"=u16 16000, "Numeric Control"=200, "y 2"=u16 65535 ("y"), "y"=u16 1000) -> ("Range"=→"Waveform Chart 2" →"Range (cm)":u16, "I2C Ref Out out"=w344:T13, "did_timeout"=→"did_timeout 2":bool, "Numeric Control 4"=→"dt 2":u32, "Array out"=w348:u16[], "array out"=w335:dbl[], "mean out"=w332:dbl, "error out"=w343:errorcluster)  [unwired: 7 in, 1 out]
    "distancaia 2" <- w332
    "mean out" <- w332
    n161 = Less?(x=w332, y="y") -> (x < y?=w330:bool)
    "objeto" <- w330
    n162 = local read "PARAR 2"() -> (w333:bool)
    n163 = local write "objeto"(w330) -> ()
  }
  n164 = call "stopContinuous.vi"("error in"=w14, "Slave Address(7 bit)"=w11, "I2C Ref In"=w15) -> ("error out"=w13:errorcluster, "I2C Ref Out"=w12:T13)  [unwired: 7 in]
  n165 = Array To Spreadsheet String(delimiter (Tab)="\n", array=w6, 3:"" ("format string")) -> (spreadsheet string=→"spreadsheet string":string)
  n166 = call <vilib>:"Close.vi"("error in (no error)"=w13, "I2C Ref In"=w12) -> ("error out"=→"error out 2":errorcluster)  [unwired: 9 in]
  n167 = Insert Into Array(array=w52, new element #1=w51, new element #2=w43) -> (w50:T7[])  [unwired: 1 in]
  n168 = for {
    tunnel: w61 -> [w354]
    tunnel: w50 -> [w353] mode=indexing
    n169 = call <vilib>:"Close.vi"("error in (no error)"=w354, "PWM Ref In"=w353) -> ()  [unwired: 9 in, 1 out]
  }
  "indexador" <- 0
